vi "ackReportCompleteCMD.vi"(8 "error in (no error)":errorcluster, 10 "CommandValue":T1, 11 "Model in":refnum<class "Model.lvclass">) -> (0 "error out":errorcluster, 3 "Model out":refnum<class "Model.lvclass">)   [LabVIEW 2016, in "Model.lvclass"]
uses:
  Model.lvclass
  Typedefs/CommandValue.ctl
  Model.lvclass/Model.ctl
  PubSubDataEvent/PubSubDataEvent.lvclass/PubSubDataEvent.ctl
  Typedefs/SEDSpectrometerTypedefs.lvlib
  PubSubDataEvent/PubSubDataEvent.lvclass
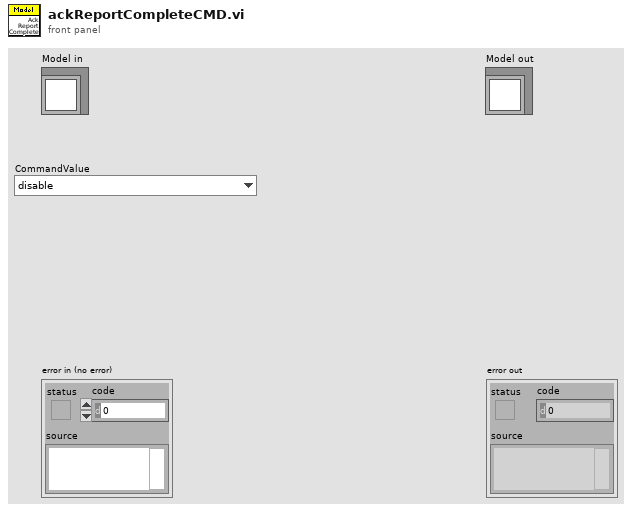
[diagram p1: front panel]
types:
  T1 = typedef "SEDSpectrometerTypedefs.lvlib/CommandValue.ctl" = enum16{"disable", "enable", "exit", "GoToStandby", "OnHeartbeat", "OnIncomingMessagingError", "OnInterrupt", "start", "captureSpectImage", "setSpectTempSetpoint", "stopImageCapture"}
  T2 = cluster{"error":i32, "result":string, "ack":i32, "cmdSeqNum":i32, "CommandValue":T1}
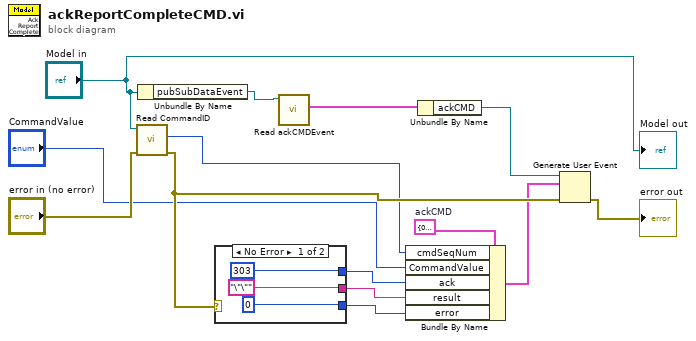
[diagram p0: block diagram]
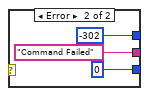
[diagram p2: hidden frame]
diagram:
  w8 = T2 {"error"=0, "result"="", "ack"=0, "cmdSeqNum"=0, "CommandValue"=enum."disable"}  # ackCMD
  n1 = call-dynamic "Read CommandID.vi"("error in (no error)"="error in (no error)", "Model in"="Model in") -> ("error out"=w7:errorcluster, "CommandID"=w1:i32)  [unwired: 7 in, 1 out]
  n2 = Unbundle By Name("Model in") -> ("pubSubDataEvent"=w10:refnum<class "PubSubDataEvent.lvclass">)
  n3 = case shown="No Error" w7 {
    tunnel: [0 ("error") 0 ("error")] -> w5
    tunnel: ["\"\"" ("result") "Command Failed" ("result")] -> w4
    tunnel: [303 ("ack") -302 ("ack")] -> w3
    frame No Error {
    }
    frame Error {
    }
  }
  n4 = call "Read ackCMDEvent.vi"("PubSubDataEvent in"=w10) -> ("ackCMDEvent"=w9:cluster{"ackCMD":refnum<user-event>})  [unwired: 8 in, 2 out]
  n5 = Bundle By Name(cluster=w8, "cmdSeqNum"=w1, "CommandValue"="CommandValue", "ack"=w3, "result"=w4, "error"=w5) -> (w6:T2)
  n6 = Unbundle By Name(w9) -> ("ackCMD"=w14:refnum<user-event>)
  n7 = Generate User Event(user event=w14, event data cluster=w6, error in=w7) -> (error out=→"error out":errorcluster)  [unwired: 1 in, 1 out]
  "Model out" <- "Model in"
